vi "lab.vi"() -> ()   [LabVIEW 2016]
uses:
  ImageBrightness.dll
panel:
  out "Result":T1(plugin-control)
  out "Original":T1(plugin-control)
  in  "Radio Buttons":enum32{"Simple", "vi", "dll", "VISION"}(radio)
  in  "Путь к изображению":path
  in  "Старт":bool
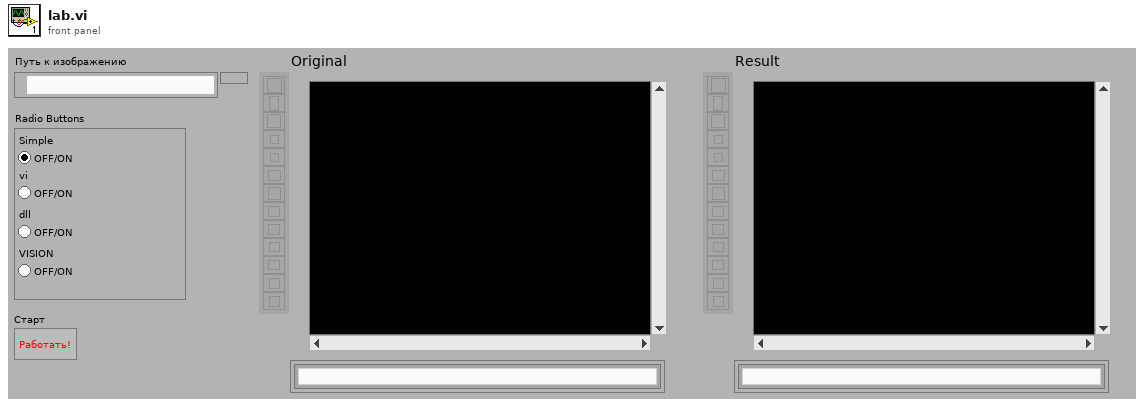
[diagram p1: front panel]
types:
  T1 = typedef "IMAQ Image.ctl" = refnum<image>
  T2 = typedef "imagedata.ctl" = cluster{"image type":i32, "image depth":i32, "image":u8[], "mask":u8[], "colors":u32[], "Rectangle":cluster{"left":i16, "top":i16, "right":i16, "bottom":i16}}
  T3 = typedef "Image Type" = u32
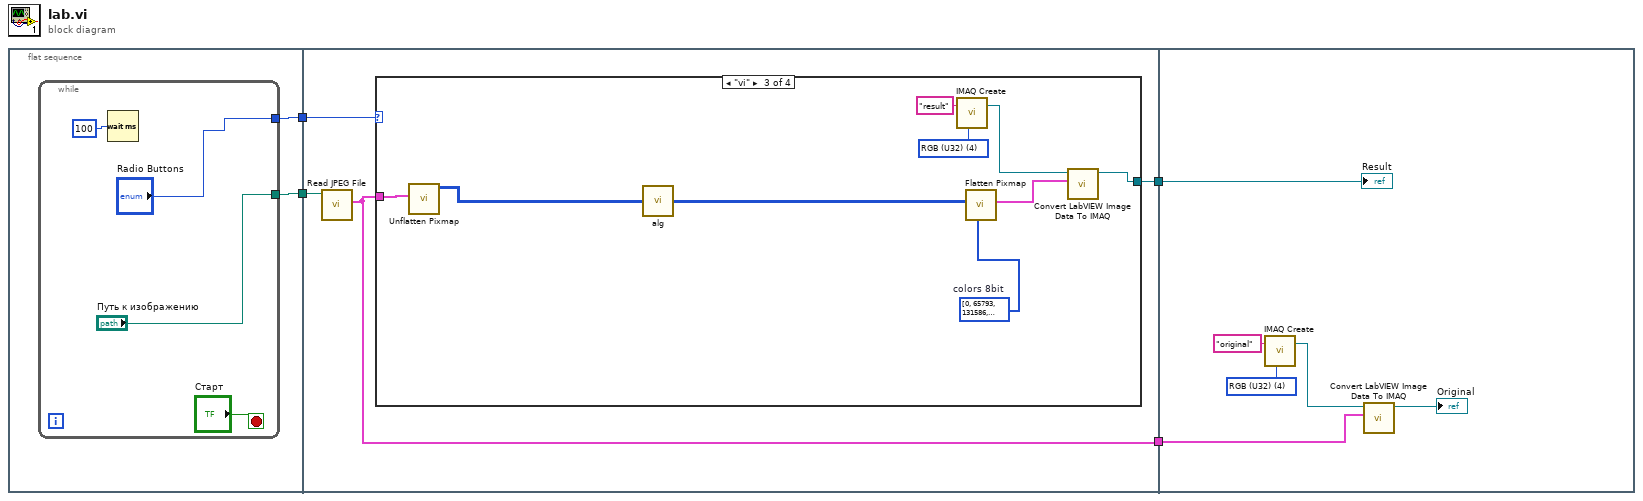
[diagram p0: block diagram]
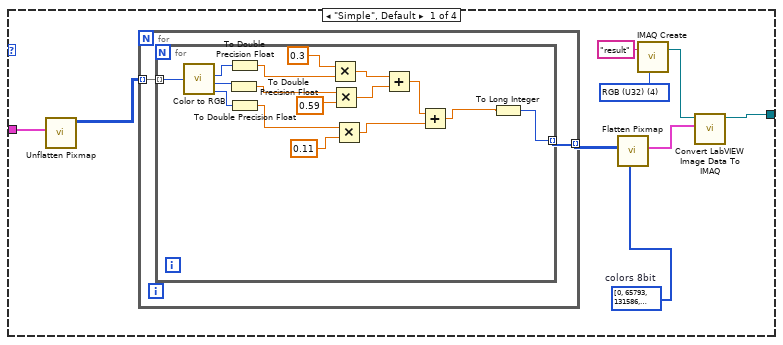
[diagram p2: hidden frame]
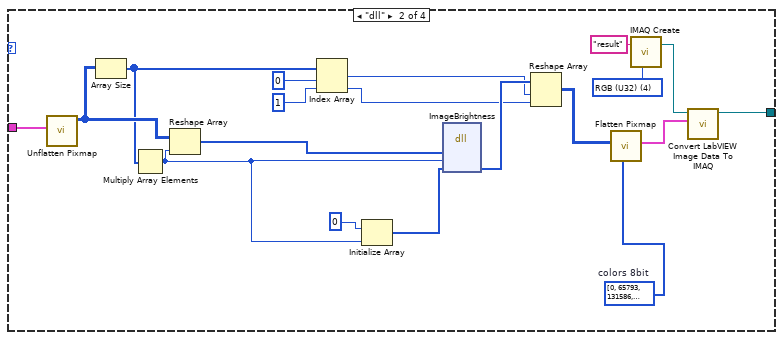
[diagram p3: hidden frame]
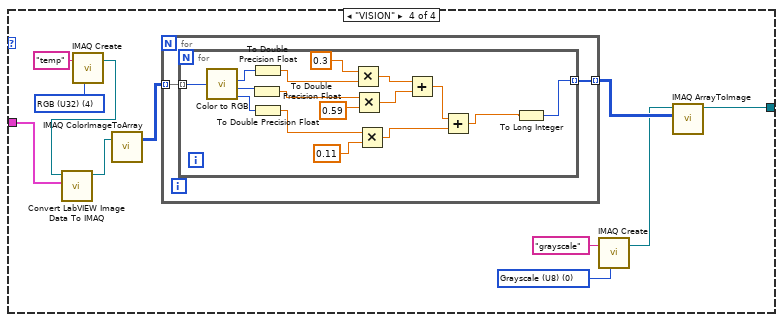
[diagram p4: hidden frame]
diagram:
  n1 = flat-sequence {
    tunnel: [w6] -> w3
    tunnel: [w5] -> w2
    tunnel: [w12] -> w4
    tunnel: w3 -> [w14]
    tunnel: w2 -> [w13]
    tunnel: [w11] -> w1
    tunnel: w4 -> [w104]
    tunnel: w1 -> [w102]
    frame #0 {
      n2 = while {
        tunnel: ["Путь к изображению"] -> w6
        tunnel: ["Radio Buttons"] -> w5
        stop <- "Старт" stop-if-true
        n3 = Wait (ms)(milliseconds to wait=100) -> ()  [unwired: 1 out]
      }
    }
    frame #1 {
      n4 = call <vilib>:"Read JPEG File.vi"("path to JPEG file"=w14) -> ("image data"=w12:T2)  [unwired: 8 in, 2 out]
      n5 = case shown="\"vi\"" w13 {
        tunnel: w12 -> [w15 w58 w69 w71]
        tunnel: [w21 w51 w65 w70] -> w11
        frame "Simple", Default {
          w18 = T3 4 items=["Grayscale (U8)", "Grayscale (I16)", "Grayscale (SGL)", "Complex (CSG)", "RGB (U32)", "HSL (U32)", "RGB (U64)", "Grayscale (U16)"] ("Image Type")
          w23 = u32[] [0, 65793, 131586, 197379, 263172, 328965, 394758, 460551, 526344, 592137, 657930, 723723, 789516, 855309, 921102, 986895, 1052688, 1118481, 1184274, 1250067, 1315860, 1381653, 1447446, 1513239, 1579032, 1644825, 1710618, 1776411, 1842204, 1907997, 1973790, 2039583, 2105376, 2171169, 2236962, 2302755, 2368548, 2434341, 2500134, 2565927, 2631720, 2697513, 2763306, 2829099, 2894892, 2960685, 3026478, 3092271, 3158064, 3223857, 3289650, 3355443, 3421236, 3487029, 3552822, 3618615, 3684408, 3750201, 3815994, 3881787, 3947580, 4013373, 4079166, 4144959, 4210752, 4276545, 4342338, 4408131, 4473924, 4539717, 4605510, 4671303, 4737096, 4802889, 4868682, 4934475, 5000268, 5066061, 5131854, 5197647, 5263440, 5329233, 5395026, 5460819, 5526612, 5592405, 5658198, 5723991, 5789784, 5855577, 5921370, 5987163, 6052956, 6118749, 6184542, 6250335, 6316128, 6381921, 6447714, 6513507, 6579300, 6645093, 6710886, 6776679, 6842472, 6908265, 6974058, 7039851, 7105644, 7171437, 7237230, 7303023, 7368816, 7434609, 7500402, 7566195, 7631988, 7697781, 7763574, 7829367, 7895160, 7960953, 8026746, 8092539, 8158332, 8224125, 8289918, 8355711, 8421504, 8487297, 8553090, 8618883, 8684676, 8750469, 8816262, 8882055, 8947848, 9013641, 9079434, 9145227, 9211020, 9276813, 9342606, 9408399, 9474192, 9539985, 9605778, 9671571, 9737364, 9803157, 9868950, 9934743, 10000536, 10066329, 10132122, 10197915, 10263708, 10329501, 10395294, 10461087, 10526880, 10592673, 10658466, 10724259, 10790052, 10855845, 10921638, 10987431, 11053224, 11119017, 11184810, 11250603, 11316396, 11382189, 11447982, 11513775, 11579568, 11645361, 11711154, 11776947, 11842740, 11908533, 11974326, 12040119, 12105912, 12171705, 12237498, 12303291, 12369084, 12434877, 12500670, 12566463, 12632256, 12698049, 12763842, 12829635, 12895428, 12961221, 13027014, 13092807, 13158600, 13224393, 13290186, 13355979, 13421772, 13487565, 13553358, 13619151, 13684944, 13750737, 13816530, 13882323, 13948116, 14013909, 14079702, 14145495, 14211288, 14277081, 14342874, 14408667, 14474460, 14540253, 14606046, 14671839, 14737632, 14803425, 14869218, 14935011, 15000804, 15066597, 15132390, 15198183, 15263976, 15329769, 15395562, 15461355, 15527148, 15592941, 15658734, 15724527, 15790320, 15856113, 15921906, 15987699, 16053492, 16119285, 16185078, 16250871, 16316664, 16382457, 16448250, 16514043, 16579836, 16645629, 16711422, 16777215]  # colors 8bit
          n6 = call <vilib>:"Unflatten Pixmap.vi"("image data"=w15) -> ("24-bit pixmap"=w16:u32[][])  [unwired: 4 in, 6 out]
          n7 = for {
            tunnel: w16 -> [w25] mode=indexing
            tunnel: [w24] -> w22 mode=indexing
            n8 = for {
              tunnel: w25 -> [w41] mode=indexing
              tunnel: [w26] -> w24 mode=indexing
              n9 = call <vilib>:"Color to RGB.vi"("Color"=w41) -> ("R"=w33:u8, "G"=w31:u8, "B"=w29:u8)  [unwired: 1 out]
              n10 = To Double Precision Float(number=w31) -> (double precision float=w30:dbl)
              n11 = To Double Precision Float(number=w33) -> (double precision float=w32:dbl)
              n12 = To Double Precision Float(number=w29) -> (double precision float=w28:dbl)
              n13 = Multiply(x=0.3, y=w32) -> (x*y=w37:dbl)
              n14 = Multiply(x=w30, y=0.59) -> (x*y=w36:dbl)
              n15 = Multiply(x=w28, y=0.11) -> (x*y=w35:dbl)
              n16 = Add(x=w37, y=w36) -> (x+y=w34:dbl)
              n17 = Add(x=w34, y=w35) -> (x+y=w27:dbl)
              n18 = To Long Integer(number=w27) -> (32bit integer=w26:i32)
            }
          }
          n19 = call <vilib>:"Flatten Pixmap.vi"("colors"=w23, "8-bit pixmap"=w22) -> ("image data"=w20:T2)  [unwired: 9 in]
          n20 = call "IMAQ Create"("Image Name"="result", "Image Type"=w18) -> ("New Image"=w17:T1)  [unwired: 3 in, 1 out]
          n21 = call "Convert LabVIEW Image Data To IMAQ.vi"("Image Data"=w20, "Image In"=w17) -> ("Image Out"=w21:T1)  [unwired: 8 in, 1 out]
        }
        frame "dll" {
          w53 = T3 4 items=["Grayscale (U8)", "Grayscale (I16)", "Grayscale (SGL)", "Complex (CSG)", "RGB (U32)", "HSL (U32)", "RGB (U64)", "Grayscale (U16)"] ("Image Type")
          w56 = u32[] [0, 65793, 131586, 197379, 263172, 328965, 394758, 460551, 526344, 592137, 657930, 723723, 789516, 855309, 921102, 986895, 1052688, 1118481, 1184274, 1250067, 1315860, 1381653, 1447446, 1513239, 1579032, 1644825, 1710618, 1776411, 1842204, 1907997, 1973790, 2039583, 2105376, 2171169, 2236962, 2302755, 2368548, 2434341, 2500134, 2565927, 2631720, 2697513, 2763306, 2829099, 2894892, 2960685, 3026478, 3092271, 3158064, 3223857, 3289650, 3355443, 3421236, 3487029, 3552822, 3618615, 3684408, 3750201, 3815994, 3881787, 3947580, 4013373, 4079166, 4144959, 4210752, 4276545, 4342338, 4408131, 4473924, 4539717, 4605510, 4671303, 4737096, 4802889, 4868682, 4934475, 5000268, 5066061, 5131854, 5197647, 5263440, 5329233, 5395026, 5460819, 5526612, 5592405, 5658198, 5723991, 5789784, 5855577, 5921370, 5987163, 6052956, 6118749, 6184542, 6250335, 6316128, 6381921, 6447714, 6513507, 6579300, 6645093, 6710886, 6776679, 6842472, 6908265, 6974058, 7039851, 7105644, 7171437, 7237230, 7303023, 7368816, 7434609, 7500402, 7566195, 7631988, 7697781, 7763574, 7829367, 7895160, 7960953, 8026746, 8092539, 8158332, 8224125, 8289918, 8355711, 8421504, 8487297, 8553090, 8618883, 8684676, 8750469, 8816262, 8882055, 8947848, 9013641, 9079434, 9145227, 9211020, 9276813, 9342606, 9408399, 9474192, 9539985, 9605778, 9671571, 9737364, 9803157, 9868950, 9934743, 10000536, 10066329, 10132122, 10197915, 10263708, 10329501, 10395294, 10461087, 10526880, 10592673, 10658466, 10724259, 10790052, 10855845, 10921638, 10987431, 11053224, 11119017, 11184810, 11250603, 11316396, 11382189, 11447982, 11513775, 11579568, 11645361, 11711154, 11776947, 11842740, 11908533, 11974326, 12040119, 12105912, 12171705, 12237498, 12303291, 12369084, 12434877, 12500670, 12566463, 12632256, 12698049, 12763842, 12829635, 12895428, 12961221, 13027014, 13092807, 13158600, 13224393, 13290186, 13355979, 13421772, 13487565, 13553358, 13619151, 13684944, 13750737, 13816530, 13882323, 13948116, 14013909, 14079702, 14145495, 14211288, 14277081, 14342874, 14408667, 14474460, 14540253, 14606046, 14671839, 14737632, 14803425, 14869218, 14935011, 15000804, 15066597, 15132390, 15198183, 15263976, 15329769, 15395562, 15461355, 15527148, 15592941, 15658734, 15724527, 15790320, 15856113, 15921906, 15987699, 16053492, 16119285, 16185078, 16250871, 16316664, 16382457, 16448250, 16514043, 16579836, 16645629, 16711422, 16777215]  # colors 8bit
          n22 = call <vilib>:"Unflatten Pixmap.vi"("image data"=w58) -> ("24-bit pixmap"=w45:u32[][])  [unwired: 4 in, 6 out]
          n23 = Array Size(array=w45) -> (size(s)=w42:i32[])
          n24 = Multiply Array Elements(1:w42) -> (0:w43:i32)
          n25 = Reshape Array(w45, w43) -> (w57:u32[])
          n26 = Index Array(array=w42, index #1=0 ("index"), index #2=1 ("index")) -> (element #1=w44:i32, element #2=w47:i32)
          n27 = Initialize Array(0 ("size(s)"), w43) -> (w59:i32[])
          n28 = dll-call lib="D:/Sources/APGS/ImageBrightness.dll" fn="ImageBrightness"("inputData"=w57, "num"=w43, "result"=w59) -> ("result"=w49:u8[])  [unwired: 6 in, 2 out]
          n29 = Reshape Array(w49, w44, w47) -> (w50:u8[][])
          n30 = call <vilib>:"Flatten Pixmap.vi"("colors"=w56, "8-bit pixmap"=w50) -> ("image data"=w55:T2)  [unwired: 9 in]
          n31 = call "IMAQ Create"("Image Name"="result", "Image Type"=w53) -> ("New Image"=w52:T1)  [unwired: 3 in, 1 out]
          n32 = call "Convert LabVIEW Image Data To IMAQ.vi"("Image Data"=w55, "Image In"=w52) -> ("Image Out"=w51:T1)  [unwired: 8 in, 1 out]
        }
        frame "vi" {
          w62 = T3 4 items=["Grayscale (U8)", "Grayscale (I16)", "Grayscale (SGL)", "Complex (CSG)", "RGB (U32)", "HSL (U32)", "RGB (U64)", "Grayscale (U16)"] ("Image Type")
          w67 = u32[] [0, 65793, 131586, 197379, 263172, 328965, 394758, 460551, 526344, 592137, 657930, 723723, 789516, 855309, 921102, 986895, 1052688, 1118481, 1184274, 1250067, 1315860, 1381653, 1447446, 1513239, 1579032, 1644825, 1710618, 1776411, 1842204, 1907997, 1973790, 2039583, 2105376, 2171169, 2236962, 2302755, 2368548, 2434341, 2500134, 2565927, 2631720, 2697513, 2763306, 2829099, 2894892, 2960685, 3026478, 3092271, 3158064, 3223857, 3289650, 3355443, 3421236, 3487029, 3552822, 3618615, 3684408, 3750201, 3815994, 3881787, 3947580, 4013373, 4079166, 4144959, 4210752, 4276545, 4342338, 4408131, 4473924, 4539717, 4605510, 4671303, 4737096, 4802889, 4868682, 4934475, 5000268, 5066061, 5131854, 5197647, 5263440, 5329233, 5395026, 5460819, 5526612, 5592405, 5658198, 5723991, 5789784, 5855577, 5921370, 5987163, 6052956, 6118749, 6184542, 6250335, 6316128, 6381921, 6447714, 6513507, 6579300, 6645093, 6710886, 6776679, 6842472, 6908265, 6974058, 7039851, 7105644, 7171437, 7237230, 7303023, 7368816, 7434609, 7500402, 7566195, 7631988, 7697781, 7763574, 7829367, 7895160, 7960953, 8026746, 8092539, 8158332, 8224125, 8289918, 8355711, 8421504, 8487297, 8553090, 8618883, 8684676, 8750469, 8816262, 8882055, 8947848, 9013641, 9079434, 9145227, 9211020, 9276813, 9342606, 9408399, 9474192, 9539985, 9605778, 9671571, 9737364, 9803157, 9868950, 9934743, 10000536, 10066329, 10132122, 10197915, 10263708, 10329501, 10395294, 10461087, 10526880, 10592673, 10658466, 10724259, 10790052, 10855845, 10921638, 10987431, 11053224, 11119017, 11184810, 11250603, 11316396, 11382189, 11447982, 11513775, 11579568, 11645361, 11711154, 11776947, 11842740, 11908533, 11974326, 12040119, 12105912, 12171705, 12237498, 12303291, 12369084, 12434877, 12500670, 12566463, 12632256, 12698049, 12763842, 12829635, 12895428, 12961221, 13027014, 13092807, 13158600, 13224393, 13290186, 13355979, 13421772, 13487565, 13553358, 13619151, 13684944, 13750737, 13816530, 13882323, 13948116, 14013909, 14079702, 14145495, 14211288, 14277081, 14342874, 14408667, 14474460, 14540253, 14606046, 14671839, 14737632, 14803425, 14869218, 14935011, 15000804, 15066597, 15132390, 15198183, 15263976, 15329769, 15395562, 15461355, 15527148, 15592941, 15658734, 15724527, 15790320, 15856113, 15921906, 15987699, 16053492, 16119285, 16185078, 16250871, 16316664, 16382457, 16448250, 16514043, 16579836, 16645629, 16711422, 16777215]  # colors 8bit
          n33 = call <vilib>:"Unflatten Pixmap.vi"("image data"=w69) -> ("24-bit pixmap"=w68:u32[][])  [unwired: 4 in, 6 out]
          n34 = call "alg.vi"("24-bit pixmap"=w68) -> ("Array 2"=w66:i32[][])
          n35 = call "IMAQ Create"("Image Name"="result", "Image Type"=w62) -> ("New Image"=w61:T1)  [unwired: 3 in, 1 out]
          n36 = call <vilib>:"Flatten Pixmap.vi"("colors"=w67, "8-bit pixmap"=w66) -> ("image data"=w64:T2)  [unwired: 9 in]
          n37 = call "Convert LabVIEW Image Data To IMAQ.vi"("Image Data"=w64, "Image In"=w61) -> ("Image Out"=w65:T1)  [unwired: 8 in, 1 out]
        }
        frame "VISION" {
          w73 = T3 0 items=["Grayscale (U8)", "Grayscale (I16)", "Grayscale (SGL)", "Complex (CSG)", "RGB (U32)", "HSL (U32)", "RGB (U64)", "Grayscale (U16)"] ("Image Type")
          w79 = T3 4 items=["Grayscale (U8)", "Grayscale (I16)", "Grayscale (SGL)", "Complex (CSG)", "RGB (U32)", "HSL (U32)", "RGB (U64)", "Grayscale (U16)"] ("Image Type")
          n38 = call "IMAQ Create"("Image Name"="temp", "Image Type"=w79) -> ("New Image"=w78:T1)  [unwired: 3 in, 1 out]
          n39 = call "Convert LabVIEW Image Data To IMAQ.vi"("Image Data"=w71, "Image In"=w78) -> ("Image Out"=w75:T1)  [unwired: 8 in, 1 out]
          n40 = call "IMAQ ColorImageToArray"("Image"=w75) -> ("Image Pixels (U32)"=w77:u32[][])  [unwired: 3 in, 2 out]
          n41 = for {
            tunnel: w77 -> [w82] mode=indexing
            tunnel: [w81] -> w76 mode=indexing
            n42 = for {
              tunnel: w82 -> [w98] mode=indexing
              tunnel: [w83] -> w81 mode=indexing
              n43 = call <vilib>:"Color to RGB.vi"("Color"=w98) -> ("R"=w90:u8, "G"=w88:u8, "B"=w86:u8)  [unwired: 1 out]
              n44 = To Double Precision Float(number=w88) -> (double precision float=w87:dbl)
              n45 = To Double Precision Float(number=w90) -> (double precision float=w89:dbl)
              n46 = To Double Precision Float(number=w86) -> (double precision float=w85:dbl)
              n47 = Multiply(x=0.3, y=w89) -> (x*y=w94:dbl)
              n48 = Multiply(x=w87, y=0.59) -> (x*y=w93:dbl)
              n49 = Multiply(x=w85, y=0.11) -> (x*y=w92:dbl)
              n50 = Add(x=w94, y=w93) -> (x+y=w91:dbl)
              n51 = Add(x=w91, y=w92) -> (x+y=w84:dbl)
              n52 = To Long Integer(number=w84) -> (32bit integer=w83:i32)
            }
          }
          n53 = call "IMAQ Create"("Image Name"="grayscale", "Image Type"=w73) -> ("New Image"=w72:T1)  [unwired: 3 in, 1 out]
          n54 = call "IMAQ ArrayToImage"("Image Pixels (U8)"=w76, "Image"=w72) -> ("Image Out"=w70:T1)  [unwired: 8 in, 1 out]
        }
      }
    }
    frame #2 {
      w100 = T3 4 items=["Grayscale (U8)", "Grayscale (I16)", "Grayscale (SGL)", "Complex (CSG)", "RGB (U32)", "HSL (U32)", "RGB (U64)", "Grayscale (U16)"] ("Image Type")
      n55 = call "IMAQ Create"("Image Name"="original", "Image Type"=w100) -> ("New Image"=w99:T1)  [unwired: 3 in, 1 out]
      n56 = call "Convert LabVIEW Image Data To IMAQ.vi"("Image Data"=w104, "Image In"=w99) -> ("Image Out"=→"Original":T1)  [unwired: 8 in, 1 out]
      "Result" <- w102
    }
  }
